vi "Get Relative Path_Doc.vi"(8 "Error In":errorcluster, 10 "Relative Path Root":path, 11 "File / Folder":path) -> (0 "Error Out":errorcluster, 2 "Relative Path":path, 3 "Duplicate File / Folder":path)   [LabVIEW 2011, in "LVH-Toolbox.lvlib" / "LVH-Documentation.lvlib"]
doc: "Given a file or folder path and a root path, this VI returns the relative path from the root path to the file or folder path."
uses:
  LVH-Documentation.lvlib
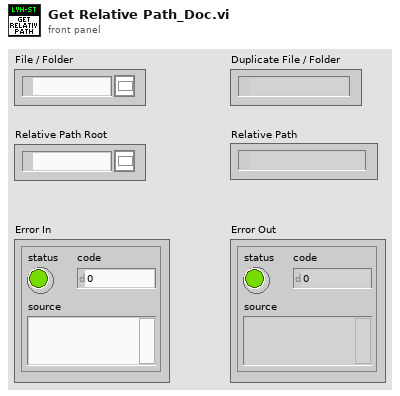
[diagram p1: front panel]
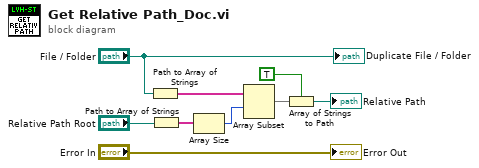
[diagram p0: block diagram]
diagram:
  n1 = Path to Array of Strings(0:"File / Folder") -> (2:w6:string[])  [unwired: 1 out]
  n2 = Path to Array of Strings(0:"Relative Path Root") -> (2:w7:string[])  [unwired: 1 out]
  n3 = Array Size(array=w7) -> (size(s)=w5:i32)
  n4 = Array Subset(array=w6, index=w5) -> (w4:string[])  [unwired: 1 in]
  n5 = Array of Strings to Path(0:w4, 1:TRUE ("relative")) -> (2:→"Relative Path":path)
  "Error Out" <- "Error In"
  "Duplicate File / Folder" <- "File / Folder"
